vi "Router - PXImc Connect.vi"(8 "error in (no error)":errorcluster, 11 "Router Data In":T1) -> (0 "error out":errorcluster, 3 "Router Data Out":T1)   [LabVIEW 2016, in "PXImc Router.lvlib"]
uses:
  PXImc Router.lvlib
  Controls/Router/Router - Config.ctl
  Controls/Router/Router - Node Block R-W Properties.ctl
  Controls/Router/Router - Block Properties.ctl
  Controls/Router/Router - PXImc Properties.ctl
  Controls/Router/Router - PXImc Card Properties.ctl
  <vilib>/pximc/Connect (U8).vi
  <vilib>/pximc/nipximc.lvlib
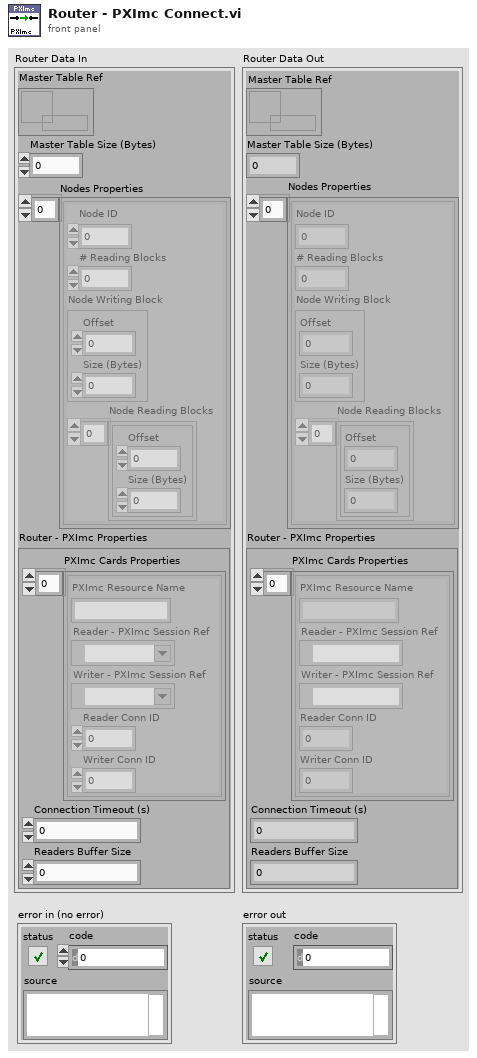
[diagram p1: front panel]
types:
  T1 = typedef "PXImc Router.lvlib/Router - Config.ctl" = cluster{"Master Table Ref":refnum<data-value>, "Master Table Size (Bytes)":u32, "Nodes Properties":T2[], "Router - PXImc Properties":T4}
  T2 = typedef "PXImc Router.lvlib/Router - Node Block R-W Properties.ctl" = cluster{"Node ID":u32, "# Reading Blocks":u32, "Node Writing Block":T3, "Node Reading Blocks":T3[]}
  T3 = typedef "PXImc Router.lvlib/Router - Block Properties.ctl" = cluster{"Offset":u32, "Size (Bytes)":u32}
  T4 = typedef "PXImc Router.lvlib/Router - PXImc Properties.ctl" = cluster{"PXImc Cards Properties":T5[], "Connection Timeout (s)":dbl, "Readers Buffer Size":u64}
  T5 = typedef "PXImc Router.lvlib/Router - PXImc Card Properties.ctl" = cluster{"PXImc Resource Name":string, "Reader - PXImc Session Ref":refnum<k21>, "Writer - PXImc Session Ref":refnum<k21>, "Reader Conn ID":u16, "Writer Conn ID":u16}
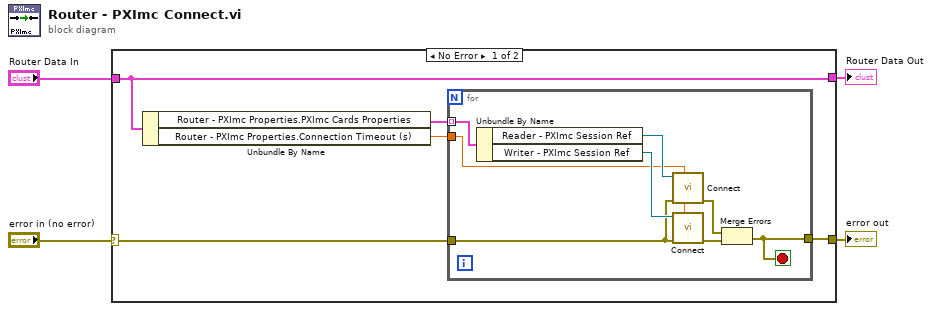
[diagram p0: block diagram]
diagram:
  n1 = case shown="No Error" "error in (no error)" {
    selector: "error in (no error)" -> [w9 w18]
    tunnel: "Router Data In" -> [w5 w19]
    tunnel: [w5 w19] -> w1
    tunnel: [w7 w18] -> w4
    frame No Error {
      n2 = Unbundle By Name(w5) -> ("Router - PXImc Properties.PXImc Cards Properties"=w8:T5[], "Router - PXImc Properties.Connection Timeout (s)"=w6:dbl)
      n3 = for {
        tunnel: w8 -> [w17] mode=indexing
        tunnel: w9 -> [w12]
        tunnel: [w16] -> w7
        tunnel: w6 -> [w13]
        stop <- w16 stop-if-true
        n4 = Unbundle By Name(w17) -> ("Reader - PXImc Session Ref"=w15:refnum<k21>, "Writer - PXImc Session Ref"=w14:refnum<k21>)
        n5 = call-poly <vilib>:"Connect.vi"("timeout in seconds (-1)"=w13, "error in (no error)"=w12, "session in"=w15) -> ("error out"=w11:errorcluster)  [unwired: 7 in, 1 out]
        n6 = call-poly <vilib>:"Connect.vi"("timeout in seconds (-1)"=w13, "error in (no error)"=w12, "session in"=w14) -> ("error out"=w10:errorcluster)  [unwired: 7 in, 1 out]
        n7 = Merge Errors(w11, w10) -> (w16:errorcluster)
      }
    }
    frame Error {
    }
  }
  "error out" <- w4
  "Router Data Out" <- w1
